vi "Servo Control-780nm_WC.vi"(4 "DMD Shutter":bool=TRUE) -> ()   [LabVIEW 2016]
uses:
  C:/Program Files (x86)/National Instruments/LabVIEW 2016/examples/Instrument IO/Serial/support/Serial - Settings.ctl
  <vilib>/Instr/_visa.llb/VISA Configure Serial Port (Instr).vi
panel:
  out "Servo FLag S4":u16=15 max=15 step=1 format="%x"
  in  "Servo S4":u16=15 caption="Servo" max=15 step=1
  in  "Position S4":u16(knob)=90 caption="Position" max=180 scale=0.0..180.0
  in  "Speed S4":u16=180 caption="Speed" max=180 step=9
  in  "VISA resource name":refnum<visa-resource-name>="COM9"
  in  "Serial Settings":T1={"baud rate"=9600, "data bits"=8, "parity"=enum."None", "stop bits"=10, "flow control"=0} {"flow control" items=["None"=0, "XON/XOFF"=1, "RTS/CTS"=2, "DTR/DSR"=4]; "stop bits" items=["1.0"=10, "1.5"=15, "2.0"=20]; "data bits" min=5 max=8 step=1; "baud rate" items=["75"=75, "110"=110, "134"=134, "150"=150, "300"=300, "600"=600, "1200"=1200, "1800"=1800, "2400"=2400, "4800"=4800, "7200"=7200, "9600"=9600, "14400"=14400, "19200"=19200, "28800"=28800, "38400"=38400, "56000"=56000, "57600"=57600, "115200"=115200, "128000"=128000, "230400"=230400]}
  in  "Command":string="ÿ\u0002\fw\u0007ÿ\u0002\rn\u0002ÿ\u0002\u000e5\u0006ÿ\u0002\u000fÜ\u0005"
  # "Servo 4(DMD)"
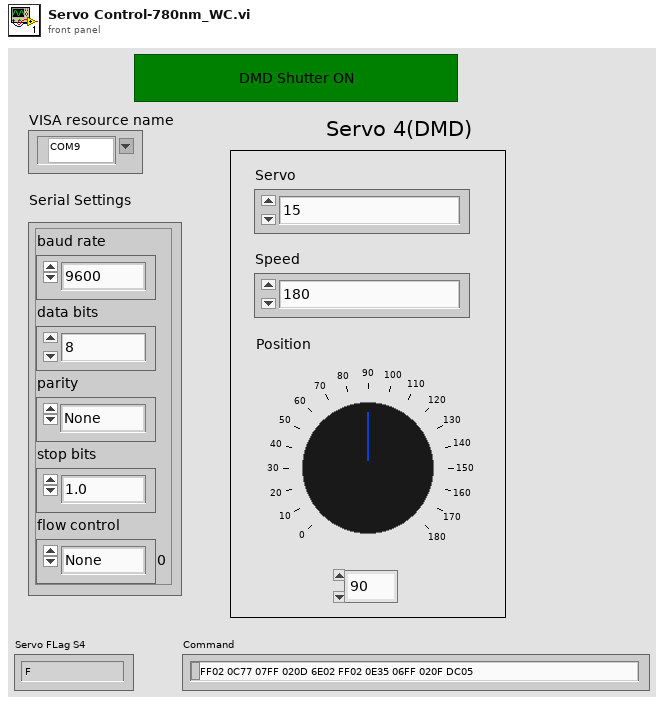
[diagram p1: front panel]
types:
  T1 = typedef "Serial - Settings.ctl" = cluster{"baud rate":u32, "data bits":u16, "parity":enum16{"None", "Odd", "Even", "Mark", "Space"}, "stop bits":u16, "flow control":u16}
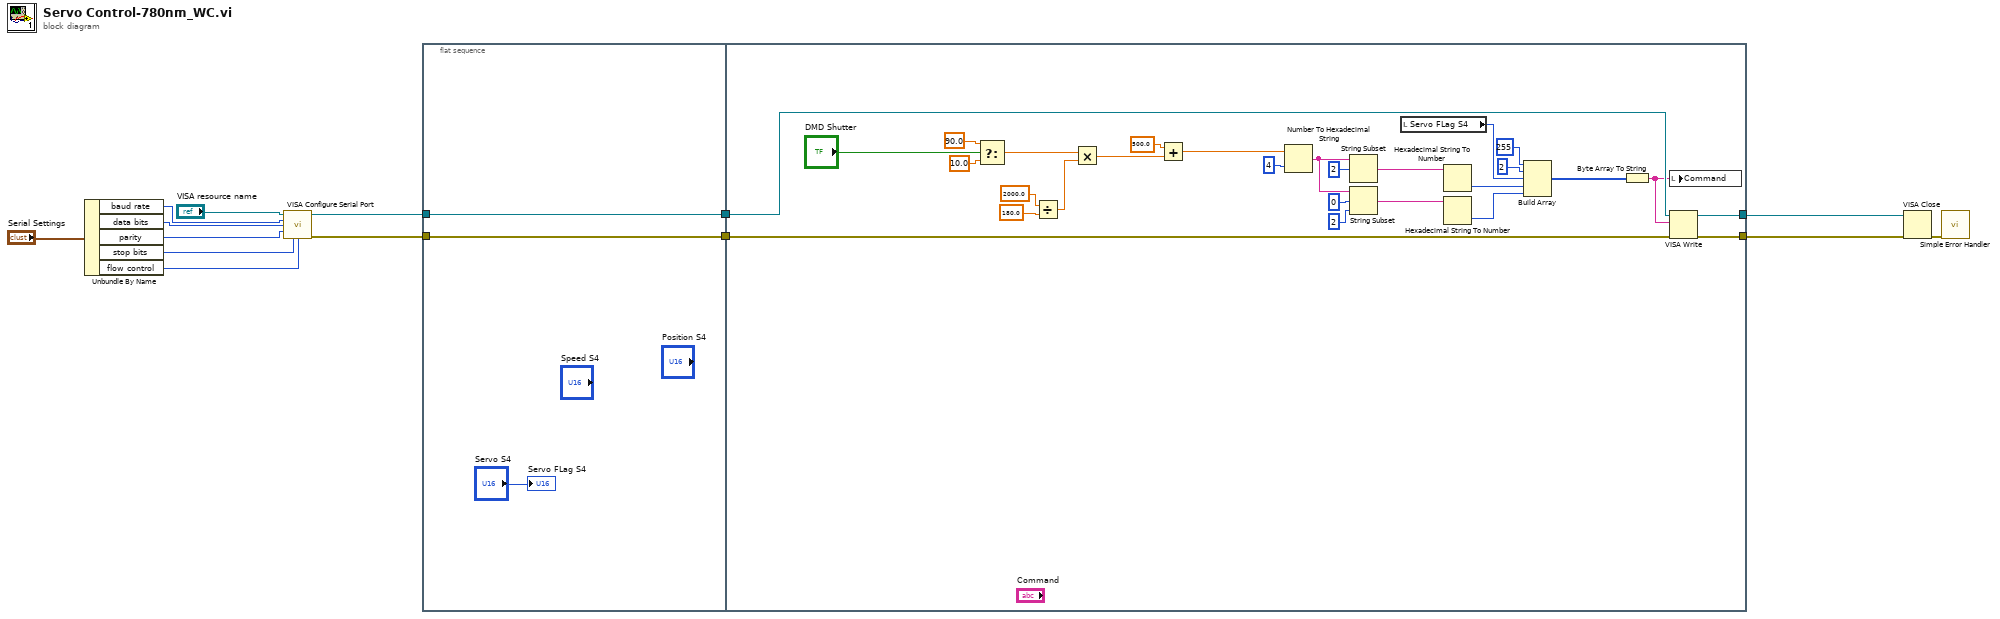
[diagram p0: block diagram]
diagram:
  n1 = Unbundle By Name("Serial Settings") -> ("baud rate"=w10:u32, "data bits"=w11:u16, "parity"=w12:enum16{"None", "Odd", "Even", "Mark", "Space"}, "stop bits"=w13:u16, "flow control"=w8:u16)
  n2 = call-poly "VISA Configure Serial Port"("VISA resource name"="VISA resource name", "baud rate (9600)"=w10, "data bits (8)"=w11, "parity (0:none)"=w12, "stop bits (10: 1 bit)"=w13, "flow control (0:none)"=w8) -> ("VISA resource name out"=w7:refnum<visa-resource-name>, "error out"=w6:errorcluster)  [unwired: 4 in, 4 out]
  n3 = flat-sequence {
    tunnel: w6 -> [w16]
    tunnel: w7 -> [w17]
    tunnel: [w17] -> w2
    tunnel: [w16] -> w1
    tunnel: [w43] -> w4
    tunnel: [w42] -> w3
    tunnel: w2 -> [w45]
    tunnel: w1 -> [w44]
    frame #0 {
      "Servo FLag S4" <- "Servo S4"
    }
    frame #1 {
      n4 = Select(t=90.0, s="DMD Shutter", f=10.0) -> (s? t:f=w19:dbl)
      n5 = Divide(x=2000.0, y=180.0) -> (x/y=w34:dbl)
      n6 = Multiply(x=w19, y=w34) -> (x*y=w33:dbl)
      n7 = Add(x=500.0, y=w33) -> (x+y=w24:dbl)
      n8 = Number To Hexadecimal String(1:i16 4 ("width (-)"), 2:w24) -> (0:w28:string)
      n9 = String Subset(string=w28, offset (0)=2) -> (substring=w27:string)  [unwired: 1 in]
      n10 = String Subset(string=w28, offset (0)=0, length (rest)=2 ("length (rest)")) -> (substring=w26:string)
      n11 = local read "Servo FLag S4"() -> (w37:u16)
      n12 = Hexadecimal String To Number(string=w27) -> (number=w23:u32)  [unwired: 2 in, 1 out]
      n13 = Hexadecimal String To Number(string=w26) -> (number=w18:u32)  [unwired: 2 in, 1 out]
      n14 = Build Array(255, 2, w37, w23, w18) -> (w40:u32[])
      n15 = Byte Array To String(unsigned byte array=w40) -> (string=w41:string)
      n16 = local write "Command"(w41) -> ()
      n17 = VISA Write(VISA resource name=w45, write buffer=w41, error in (no error)=w44) -> (VISA resource name out=w43:refnum<visa-resource-name>, error out=w42:errorcluster)  [unwired: 1 out]
    }
  }
  n18 = VISA Close(VISA resource name=w4, error in (no error)=w3) -> (error out=w5:errorcluster)
  n19 = call <vilib>:"Simple Error Handler.vi"("error in (no error)"=w5) -> ()  [unwired: 1 in, 8 out]
